vi "Execute Function.vi"(8 "error in (no error)":errorcluster, 10 "Modbus request":refnum<class "Modbus Data Unit (PDU).lvclass">, 11 "device data model in":refnum<class "Standard Data Model.lvclass">) -> (0 "error out":errorcluster, 2 "Modbus response":refnum<class "Modbus Data Unit (PDU).lvclass">, 3 "device data model out":refnum<class "Standard Data Model.lvclass">)   [LabVIEW 2015, in "SubVIs.lvlib" / "Standard Data Model.lvclass"]
doc: "This function is responsible for deciding what code to execute when a specific function is called."
uses:
  <vilib>/Modbus/subvis/Data and Functions/Standard Data Model/Standard Data Model.lvclass
  <vilib>/Modbus/subvis/Modbus Data Unit (PDU)/Modbus Data Unit (PDU).lvclass
  <vilib>/Modbus/subvis/Modbus Data Unit (PDU)/Modbus Data Unit (PDU).lvclass/Modbus Data Unit (PDU).ctl
  <vilib>/Modbus/subvis/Utility/Bits to Bytes.vi
  <vilib>/Modbus/subvis/Utility/Bytes to Bits.vi
  <vilib>/Modbus/subvis/Utility/U16s to Bytes.vi
  <vilib>/Modbus/subvis/Utility/Bytes to U16s.vi
  <vilib>/Modbus/subvis/Data and Functions/Device Data Model/Access Functions/helpers/Validate Device ID Code.vi
  <vilib>/Modbus/subvis/Data and Functions/Device Data Model/Access Functions/helpers/Search Object List.vi
  <vilib>/Modbus/subvis/Data and Functions/Device Data Model/Access Functions/helpers/Process Objects.vi
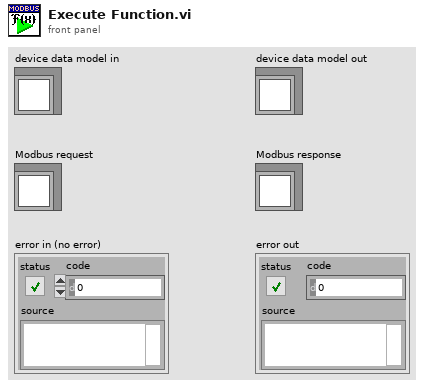
[diagram p1: front panel]
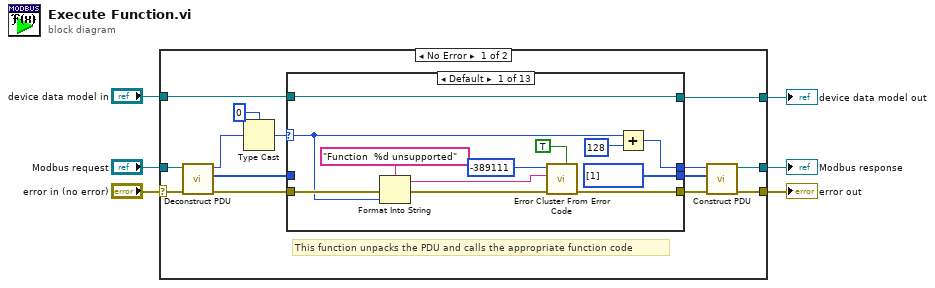
[diagram p0: block diagram]
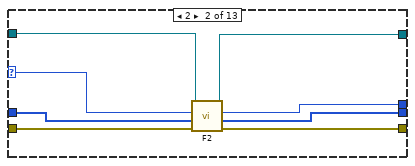
[diagram p2: hidden frame]
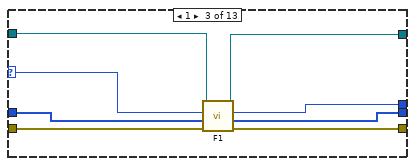
[diagram p3: hidden frame]
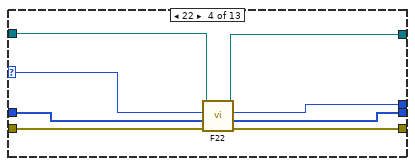
[diagram p4: hidden frame]
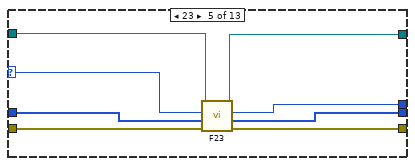
[diagram p5: hidden frame]
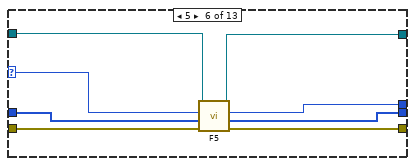
[diagram p6: hidden frame]
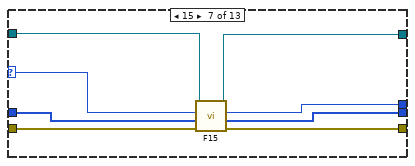
[diagram p7: hidden frame]
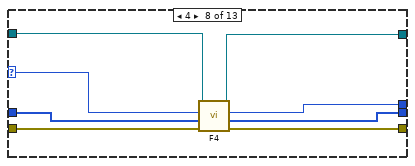
[diagram p8: hidden frame]
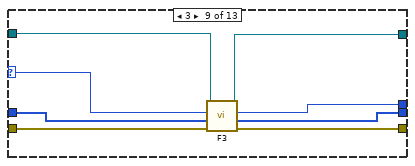
[diagram p9: hidden frame]
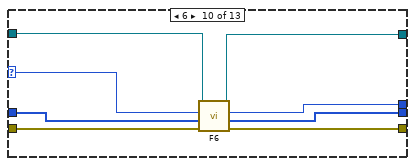
[diagram p10: hidden frame]
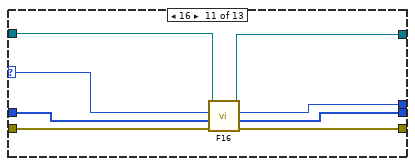
[diagram p11: hidden frame]
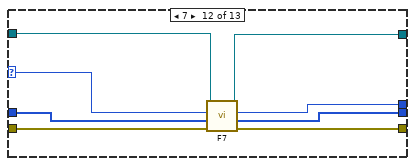
[diagram p12: hidden frame]
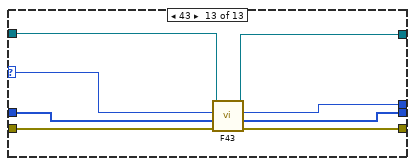
[diagram p13: hidden frame]
diagram:
  n1 = case shown="No Error" "error in (no error)" {
    selector: "error in (no error)" -> [w7 w130]
    tunnel: "device data model in" -> [w20 w129]
    tunnel: [w19 w129] -> w5
    tunnel: "Modbus request" -> [w18 w131]
    tunnel: [w13 w131] -> w3
    tunnel: [w12 w130] -> w2
    frame No Error {
      # "This function unpacks the PDU and calls the appropriate function code"
      n2 = call <vilib>:"Deconstruct PDU.vi"("error in (no error)"=w7, "Modbus data unit in"=w18) -> ("error out"=w11:errorcluster, "data"=w17:u8[], "function"=w10:u8)  [unwired: 7 in]
      n3 = Type Cast(type=u8 0, x=w10) -> (*(type *) &x=w9:u8)
      n4 = case shown="Default" w9 {
        selector: w9 -> [w21 w39 w45 w53 w61 w68 w79 w83 w95 w102 w107 w118 w121]
        tunnel: w20 -> [w22 w40 w48 w56 w64 w69 w77 w82 w96 w103 w109 w119 w124]
        tunnel: w11 -> [w27 w37 w47 w55 w63 w66 w80 w85 w94 w104 w112 w120 w128]
        tunnel: [w29 w36 w46 w54 w62 w72 w75 w86 w92 w100 w111 w114 w127] -> w16
        tunnel: w17 -> [_ w38 w44 w52 w60 w67 w78 w84 w93 w101 w108 w117 w122]
        tunnel: [w30 w34 w43 w51 w59 w70 w73 w87 w90 w98 w106 w116 w125] -> w14
        tunnel: [u8[] [1] ("Data Return") w35 w42 w50 w58 w71 w74 w88 w91 w99 w105 w115 w126] -> w15
        tunnel: [w22 w33 w41 w49 w57 w65 w76 w81 w89 w97 w110 w113 w123] -> w19
        frame Default {
          n5 = Format Into String(format string="Function  %d unsupported", error in=w27, w21) -> (resulting string=w25:string, error out=w28:errorcluster)  [unwired: 1 in]
          n6 = call <vilib>:"Error Cluster From Error Code.vi"("is warning? (False)"=TRUE, "error in (no error)"=w28, "error message (\"\")"=w25, "error code (0)"=-389111) -> ("error out"=w29:errorcluster)  [unwired: 5 in]
          n7 = Add(x=w21, y=u8 128) -> (x+y=w30:u8)
        }
        frame 2 {
          n8 = call <vilib>:"F2.vi"("error in (no error)"=w37, "data"=w38, "function"=w39, "device data model in"=w40) -> ("error out"=w36:errorcluster, "data return"=w35:u8[], "function return"=w34:u8, "device data model out"=w33:refnum<class "Standard Data Model.lvclass">)  [unwired: 4 in]
        }
        frame 1 {
          n9 = call <vilib>:"F1.vi"("error in (no error)"=w47, "data"=w44, "function"=w45, "device data model in"=w48) -> ("error out"=w46:errorcluster, "data return"=w42:u8[], "function return"=w43:u8, "device data model out"=w41:refnum<class "Standard Data Model.lvclass">)  [unwired: 4 in]
        }
        frame 22 {
          n10 = call <vilib>:"F22.vi"("error in (no error)"=w55, "data"=w52, "function"=w53, "device data model in"=w56) -> ("error out"=w54:errorcluster, "data return"=w50:u8[], "function return"=w51:u8, "device data model out"=w49:refnum<class "Standard Data Model.lvclass">)  [unwired: 4 in]
        }
        frame 23 {
          n11 = call <vilib>:"F23.vi"("error in (no error)"=w63, "data"=w60, "function"=w61, "device data model in"=w64) -> ("error out"=w62:errorcluster, "data return"=w58:u8[], "function return"=w59:u8, "device data model out"=w57:refnum<class "Standard Data Model.lvclass">)  [unwired: 4 in]
        }
        frame 5 {
          n12 = call <vilib>:"F5.vi"("error in (no error)"=w66, "data"=w67, "function"=w68, "device data model in"=w69) -> ("error out"=w72:errorcluster, "data return"=w71:u8[], "function return"=w70:u8, "device data model out"=w65:refnum<class "Standard Data Model.lvclass">)  [unwired: 4 in]
        }
        frame 15 {
          n13 = call <vilib>:"F15.vi"("error in (no error)"=w80, "data"=w78, "function"=w79, "device data model in"=w77) -> ("error out"=w75:errorcluster, "data return"=w74:u8[], "function return"=w73:u8, "device data model out"=w76:refnum<class "Standard Data Model.lvclass">)  [unwired: 4 in]
        }
        frame 4 {
          n14 = call <vilib>:"F4.vi"("error in (no error)"=w85, "data"=w84, "function"=w83, "device data model in"=w82) -> ("error out"=w86:errorcluster, "data return"=w88:u8[], "function return"=w87:u8, "device data model out"=w81:refnum<class "Standard Data Model.lvclass">)  [unwired: 4 in]
        }
        frame 3 {
          n15 = call <vilib>:"F3.vi"("error in (no error)"=w94, "data"=w93, "function"=w95, "device data model in"=w96) -> ("error out"=w92:errorcluster, "data return"=w91:u8[], "function return"=w90:u8, "device data model out"=w89:refnum<class "Standard Data Model.lvclass">)  [unwired: 4 in]
        }
        frame 6 {
          n16 = call <vilib>:"F6.vi"("error in (no error)"=w104, "data"=w101, "function"=w102, "device data model in"=w103) -> ("error out"=w100:errorcluster, "data return"=w99:u8[], "function return"=w98:u8, "device data model out"=w97:refnum<class "Standard Data Model.lvclass">)  [unwired: 4 in]
        }
        frame 16 {
          n17 = call <vilib>:"F16.vi"("error in (no error)"=w112, "data"=w108, "function"=w107, "device data model in"=w109) -> ("error out"=w111:errorcluster, "data return"=w105:u8[], "function return"=w106:u8, "device data model out"=w110:refnum<class "Standard Data Model.lvclass">)  [unwired: 4 in]
        }
        frame 7 {
          n18 = call <vilib>:"F7.vi"("error in (no error)"=w120, "data"=w117, "function"=w118, "device data model in"=w119) -> ("error out"=w114:errorcluster, "data return"=w115:u8[], "function return"=w116:u8, "device data model out"=w113:refnum<class "Standard Data Model.lvclass">)  [unwired: 4 in]
        }
        frame 43 {
          n19 = call <vilib>:"F43.vi"("error in (no error)"=w128, "data"=w122, "function"=w121, "device data model in"=w124) -> ("error out"=w127:errorcluster, "data return"=w126:u8[], "function return"=w125:u8, "device data model out"=w123:refnum<class "Standard Data Model.lvclass">)  [unwired: 4 in]
        }
      }
      n20 = call <vilib>:"Construct PDU.vi"("error in (no error)"=w16, "data"=w15, "function"=w14) -> ("error out"=w12:errorcluster, "Modbus data unit out"=w13:refnum<class "Modbus Data Unit (PDU).lvclass">)  [unwired: 7 in]
    }
    frame Error {
    }
  }
  "error out" <- w2
  "device data model out" <- w5
  "Modbus response" <- w3
